vi "11-2 UDP Sender.vi"   [LabVIEW 2014]
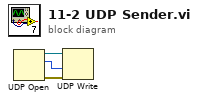
[diagram p0: block diagram]
diagram:
  n1 = UDP Open() -> (port=w1:refnum<k16>, 0:w3:errorcluster, 2:w2:u16)  [unwired: 5 in]
  n2 = UDP Write(connection ID=w1, 8:w3, 9:w2) -> ()  [unwired: 3 in, 2 out]
